vi "buffersize_test_orig.vi"() -> ()   [LabVIEW 2011]
uses:
  <vilib>/Analysis/NI_AALBase.lvlib
panel:
  out "curve & length mean":dbl[](array[numeric])
  out "wave read mean":dbl[](array[numeric])
  out "curve & length mean":dbl format="%0.2f"
  out "wave read mean":dbl format="%0.2f"
  out "overall meas time":u32
  in  "averages":i32=10
  out "external iter":i32
  out "internal iter":i32
  out "buffer sizes":i32[](array[numeric])
  out "overall meas times":dbl[](array[numeric])
  in  "buffer size start":i32
  in  "number of diff. buffer sizes":i32
  out "mean overall meas time":dbl format="%0.2f"
  out "Waveform Data":waveform(dbl)(graph)
  in  "VISA resource name":refnum<visa-resource-name>
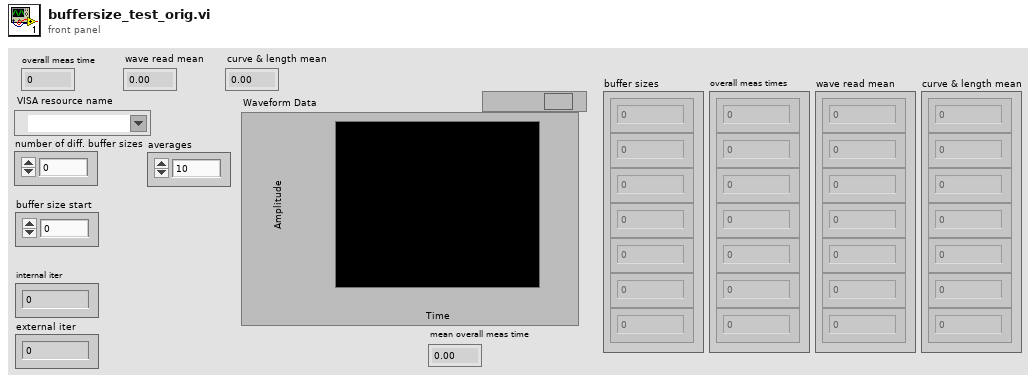
[diagram p1: front panel]
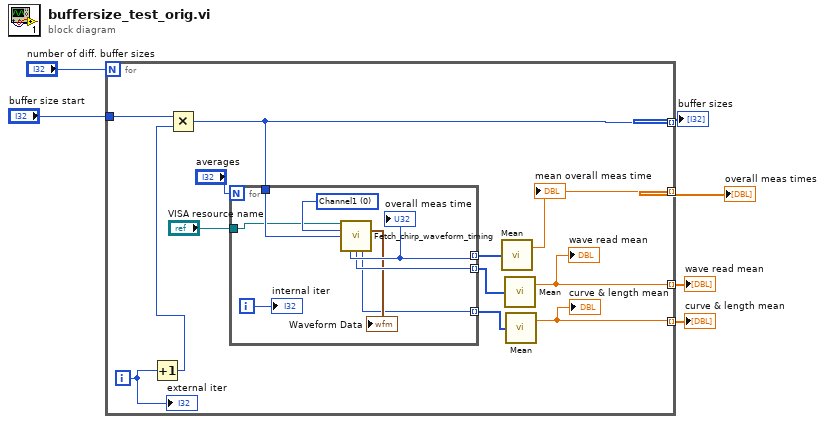
[diagram p0: block diagram]
diagram:
  n1 = for {
    N: "number of diff. buffer sizes" -> [_]
    tunnel: "buffer size start" -> [w16]
    tunnel: [w15] -> w4 mode=indexing
    tunnel: [w14] -> w3 mode=indexing
    tunnel: [w8] -> w2 mode=indexing
    tunnel: [w7] -> w1 mode=indexing
    i -> [w13]
    n2 = Increment(x=w13) -> (x+1=w12:i32)
    n3 = Multiply(x=w16, y=w12) -> (x*y=w14:i32)
    n4 = for {
      N: "averages" -> [_]
      tunnel: "VISA resource name" -> [w19]
      tunnel: w14 -> [w25]
      tunnel: [w23] -> w11 mode=indexing
      tunnel: [w22] -> w10 mode=indexing
      tunnel: [w20] -> w9 mode=indexing
      i -> [w26]
      w24 = u16 0 items=["Channel1", "Channel2", "Channel3", "Channel4", "Math1", "Math2", "Math3", "Math3", "Reference1", "Reference2", "Reference3", "Reference4"] ("Channel (0:Channel1)")
      n5 = call "Fetch_chirp_waveform_timing.vi"("VISA resource name"=w19, "Channel (0:Channel1)"=w24, "Buffer Size"=w25) -> ("Waveform Data"=→"Waveform Data":waveform(dbl), "overall meas time"=w23:u32, "read wave time"=w22:u32, "curve & length command"=w20:u32)  [unwired: 7 in, 2 out]
      "overall meas time" <- w23
      "internal iter" <- w26
    }
    n6 = call <vilib>:"Mean.vi"("X"=w11) -> ("mean"=w15:dbl)  [unwired: 1 out]
    "mean overall meas time" <- w15
    n7 = call <vilib>:"Mean.vi"("X"=w10) -> ("mean"=w8:dbl)  [unwired: 1 out]
    "wave read mean" <- w8
    n8 = call <vilib>:"Mean.vi"("X"=w9) -> ("mean"=w7:dbl)  [unwired: 1 out]
    "curve & length mean" <- w7
    "external iter" <- w13
  }
  "overall meas times" <- w4
  "buffer sizes" <- w3
  "wave read mean" <- w2
  "curve & length mean" <- w1
